vi "read until terminator.vi"(7 "Flush after read":bool=TRUE, 8 "error in (no error)":errorcluster, 9 "Timeout (ms)":i32=50, 10 "Terminator":string="\r\n", 11 "VISA Refnum in":refnum<visa-resource-name>) -> (0 "error out":errorcluster, 2 "String":string, 3 "VISA Refnum out":refnum<visa-resource-name>)   [LabVIEW 2023]
uses:
  <vilib>/Utility/error.llb/DialogType.ctl
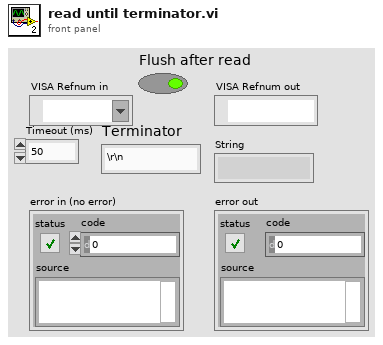
[diagram p1: front panel]
types:
  T1 = typedef "DialogType.ctl" = u16
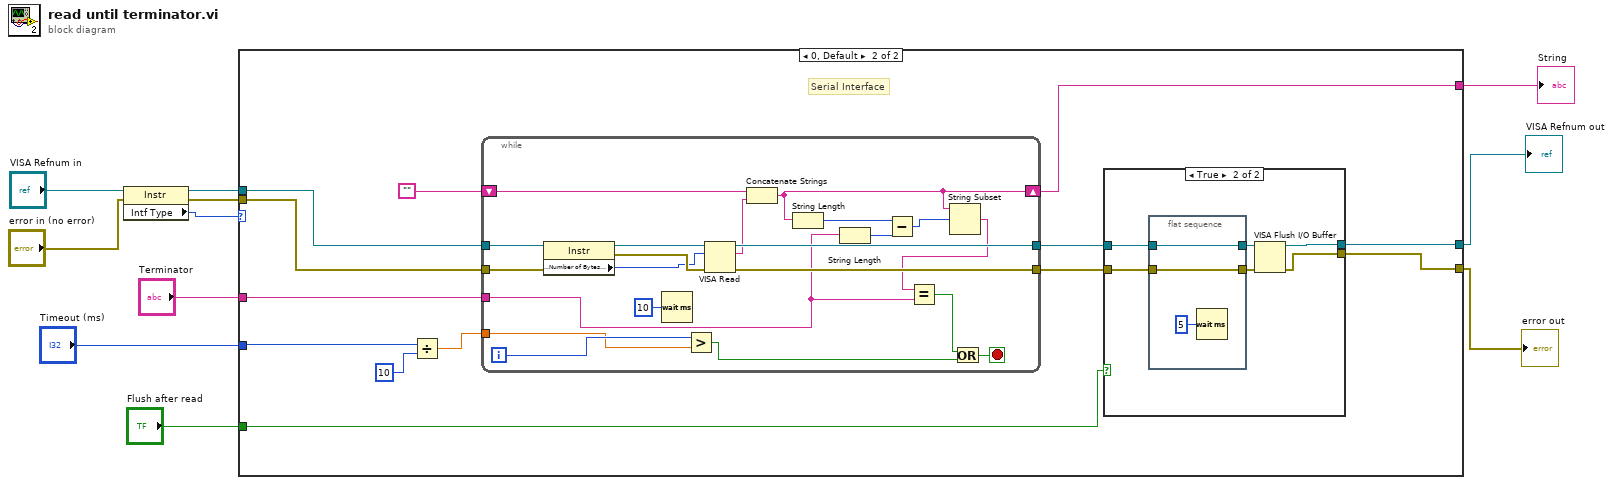
[diagram p0: block diagram]
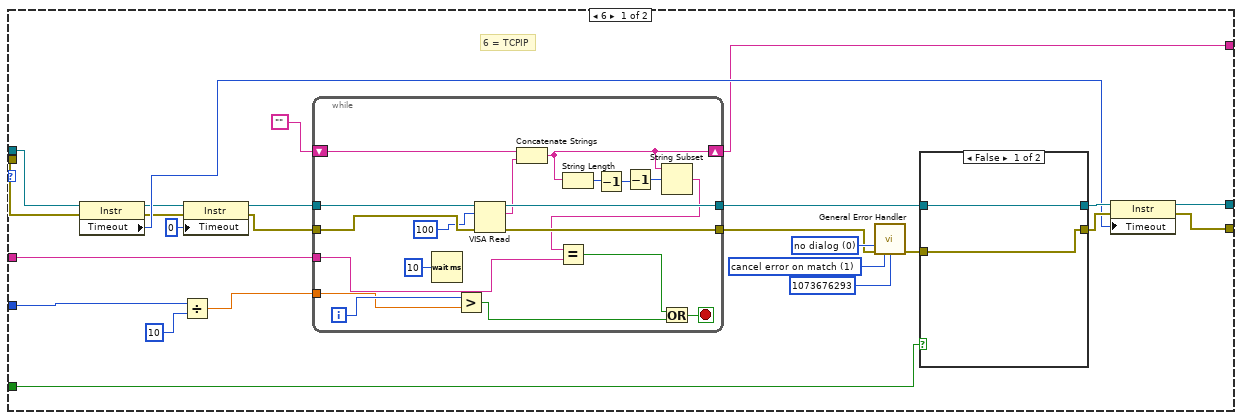
[diagram p2: hidden frame]
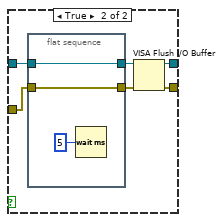
[diagram p3: hidden frame]
diagram:
  n1 = property class="Instr"(reference="VISA Refnum in", error in="error in (no error)") -> (reference out=w8:refnum<visa-resource-name>, error out=w7:errorcluster, "Intf Type"=w3:u16)
  n2 = case shown="0, Default" w3 {
    tunnel: "Terminator" -> [w34 w77]
    tunnel: w8 -> [w31 w70]
    tunnel: w7 -> [w30 w69]
    tunnel: [w25 w71] -> w6
    tunnel: [w23 w72] -> w5
    tunnel: [w14 w74] -> w4
    tunnel: "Timeout (ms)" -> [w13 w73]
    tunnel: "Flush after read" -> [w12 w67]
    frame 6 {
      w22 = T1 0 items=["no dialog", "OK message", "continue or stop message", "OK message + warnings", "continue/stop + warnings"] ("type of dialog (OK msg:1)")
      w20 = 1 items=["no exception", "cancel error on match", "set error on match"] ("[exception action] (none:0)")
      # "6 = TCPIP"
      n3 = property class="Instr"(reference=w31, error in=w30) -> (reference out=w17:refnum<visa-resource-name>, error out=w16:errorcluster, "Timeout"=w24:u32)
      n4 = Divide(x=w13, y=10) -> (x/y=w33:dbl)
      n5 = property class="Instr"(reference=w17, error in=w16, "Timeout"=u32 0 ("General Settings:Timeout Value")) -> (reference out=w29:refnum<visa-resource-name>, error out=w28:errorcluster)
      n6 = while {
        tunnel: w29 -> [w66]
        tunnel: w28 -> [w64]
        tunnel: [w65] -> w35
        tunnel: [w63] -> w19
        shift-right: [w54] -> w14
        shift-left: "" -> [w60]
        tunnel: w33 -> [w51]
        tunnel: w34 -> [w48]
        i -> [w58]
        stop <- w57 stop-if-true
        n7 = Wait (ms)(milliseconds to wait=u32 10) -> ()  [unwired: 1 out]
        n8 = Greater?(x=w58, y=w51) -> (0:w56:bool)
        n9 = VISA Read(VISA resource name=w66, byte count=u32 100 ("Bytes at Port"), error in (no error)=w64) -> (VISA resource name out=w65:refnum<visa-resource-name>, read buffer=w59:string, error out=w63:errorcluster)  [unwired: 1 out]
        n10 = Concatenate Strings(w60, w59) -> (w54:string)
        n11 = String Length(string=w54) -> (length=w55:i32)
        n12 = Decrement(x=w55) -> (x-1=w50:i32)
        n13 = Decrement(x=w50) -> (x-1=w49:i32)
        n14 = String Subset(string=w54, offset (0)=w49) -> (substring=w53:string)  [unwired: 1 in]
        n15 = Equal?(x=w53, y=w48) -> (x = y?=w52:bool)
        n16 = Or(x=w52, y=w56) -> (x .or. y?=w57:bool)
      }
      n17 = call <vilib>:"General Error Handler.vi"("type of dialog (OK msg:1)"=w22, "error in (no error)"=w19, "[exception action] (none:0)"=w20, "[exception code]"=1073676293) -> ("error out"=w18:errorcluster)  [unwired: 1 in, 10 out]
      n18 = case shown="False" w12 {
        tunnel: w35 -> [w38 w44]
        tunnel: [w38 w41] -> w27
        tunnel: [w37 w40] -> w26
        tunnel: w18 -> [w37 w39]
        frame False {
        }
        frame True {
          n19 = flat-sequence {
            tunnel: w44 -> [w46]
            tunnel: [w46] -> w43
            tunnel: w39 -> [w45]
            tunnel: [w45] -> w42
            frame #0 {
              n20 = Wait (ms)(milliseconds to wait=u32 5) -> ()  [unwired: 1 out]
            }
          }
          n21 = VISA Flush I/O Buffer(VISA resource name=w43, error in (no error)=w42) -> (VISA resource name out=w41:refnum<visa-resource-name>, error out=w40:errorcluster)  [unwired: 1 in]
        }
      }
      n22 = property class="Instr"(reference=w27, error in=w26, "Timeout"=w24) -> (reference out=w23:refnum<visa-resource-name>, error out=w25:errorcluster)
    }
    frame 0, Default {
      # "Serial Interface"
      n23 = Divide(x=w73, y=10) -> (x/y=w76:dbl)
      n24 = while {
        tunnel: w70 -> [w111]
        tunnel: w69 -> [w110]
        tunnel: [w108] -> w78
        tunnel: [w106] -> w68
        shift-right: [w98] -> w74
        shift-left: "" -> [w103]
        tunnel: w76 -> [w95]
        tunnel: w77 -> [w92]
        i -> [w101]
        stop <- w100 stop-if-true
        n25 = property class="Instr"(reference=w111, error in=w110) -> (reference out=w109:refnum<visa-resource-name>, error out=w107:errorcluster, "Serial Settings:Number of Bytes at Serial Port"=w105:u32)
        n26 = Wait (ms)(milliseconds to wait=u32 10) -> ()  [unwired: 1 out]
        n27 = Greater?(x=w101, y=w95) -> (0:w99:bool)
        n28 = VISA Read(VISA resource name=w109, byte count=w105, error in (no error)=w107) -> (VISA resource name out=w108:refnum<visa-resource-name>, read buffer=w102:string, error out=w106:errorcluster)  [unwired: 1 out]
        n29 = Concatenate Strings(w103, w102) -> (w98:string)
        n30 = String Length(string=w98) -> (length=w94:i32)
        n31 = String Length(string=w92) -> (length=w93:i32)
        n32 = Subtract(x=w94, y=w93) -> (x-y=w91:i32)
        n33 = String Subset(string=w98, offset (0)=w91) -> (substring=w97:string)  [unwired: 1 in]
        n34 = Equal?(x=w97, y=w92) -> (x = y?=w96:bool)
        n35 = Or(x=w96, y=w99) -> (x .or. y?=w100:bool)
      }
      n36 = case shown="True" w67 {
        tunnel: w78 -> [w81 w87]
        tunnel: [w81 w84] -> w72
        tunnel: [w80 w83] -> w71
        tunnel: w68 -> [w80 w82]
        frame False {
        }
        frame True {
          n37 = flat-sequence {
            tunnel: w87 -> [w89]
            tunnel: [w89] -> w86
            tunnel: w82 -> [w88]
            tunnel: [w88] -> w85
            frame #0 {
              n38 = Wait (ms)(milliseconds to wait=u32 5) -> ()  [unwired: 1 out]
            }
          }
          n39 = VISA Flush I/O Buffer(VISA resource name=w86, error in (no error)=w85) -> (VISA resource name out=w84:refnum<visa-resource-name>, error out=w83:errorcluster)  [unwired: 1 in]
        }
      }
    }
  }
  "VISA Refnum out" <- w5
  "error out" <- w6
  "String" <- w4
